vi "test New And Old Values Match.vi"(8 "error in (no error)":errorcluster, 11 "TestCase in":refnum<class "Routing and Faulting State Value Table Unit Tests.lvclass">) -> (0 "error out":errorcluster, 3 "TestCase out":refnum<class "Routing and Faulting State Value Table Unit Tests.lvclass">)   [LabVIEW 2019, in "Routing and Faulting State Value Table Unit Tests.lvclass"]
uses:
  Routing and Faulting State Value Table Unit Tests.lvclass
  Shared/Channel States.ctl
  Shared/Routing State.ctl
  Shared/Connection.ctl
  System Explorer/State-Value Row.ctl
  Routing and Faulting State Value Table Unit Tests.lvclass/Routing and Faulting State Value Table Unit Tests.ctl
  <vilib>/addons/_JKI Toolkits/VI Tester/TestCase.llb/TestCase.lvclass
  System Explorer/Routing and Faulting System Explorer.lvlib
  Shared/Routing and Faulting Shared.lvlib
  Scripting/Routing and Faulting Scripting.lvlib
  C:/Program Files (x86)/National Instruments/LabVIEW 2019/vi.lib/addons/_JKI Toolkits/VI Tester/TestCase.llb/TestCase.lvclass
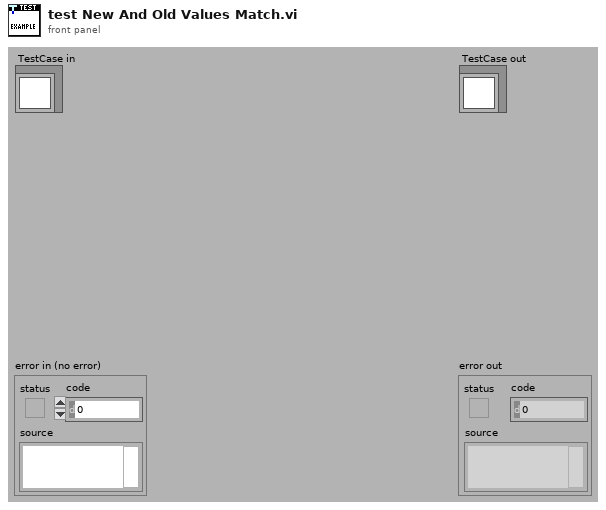
[diagram p1: front panel]
types:
  T1 = typedef "Routing and Faulting System Explorer.lvlib/State-Value Row.ctl" = cluster{"State":string, "State Value":string}
  T2 = typedef "Routing and Faulting Shared.lvlib/Channel States.ctl" = T3[]
  T3 = typedef "Routing and Faulting Shared.lvlib/Routing State.ctl" = cluster{"Name":string, "Description":string, "Value":i32, "Connection List":T4[]}
  T4 = typedef "Routing and Faulting Shared.lvlib/Connection.ctl" = cluster{"Module":string, "Source":string, "Destination":string}
  T5 = typedef "Custom Device API.lvlib/Custom Device Item Ref.ctl" = u64
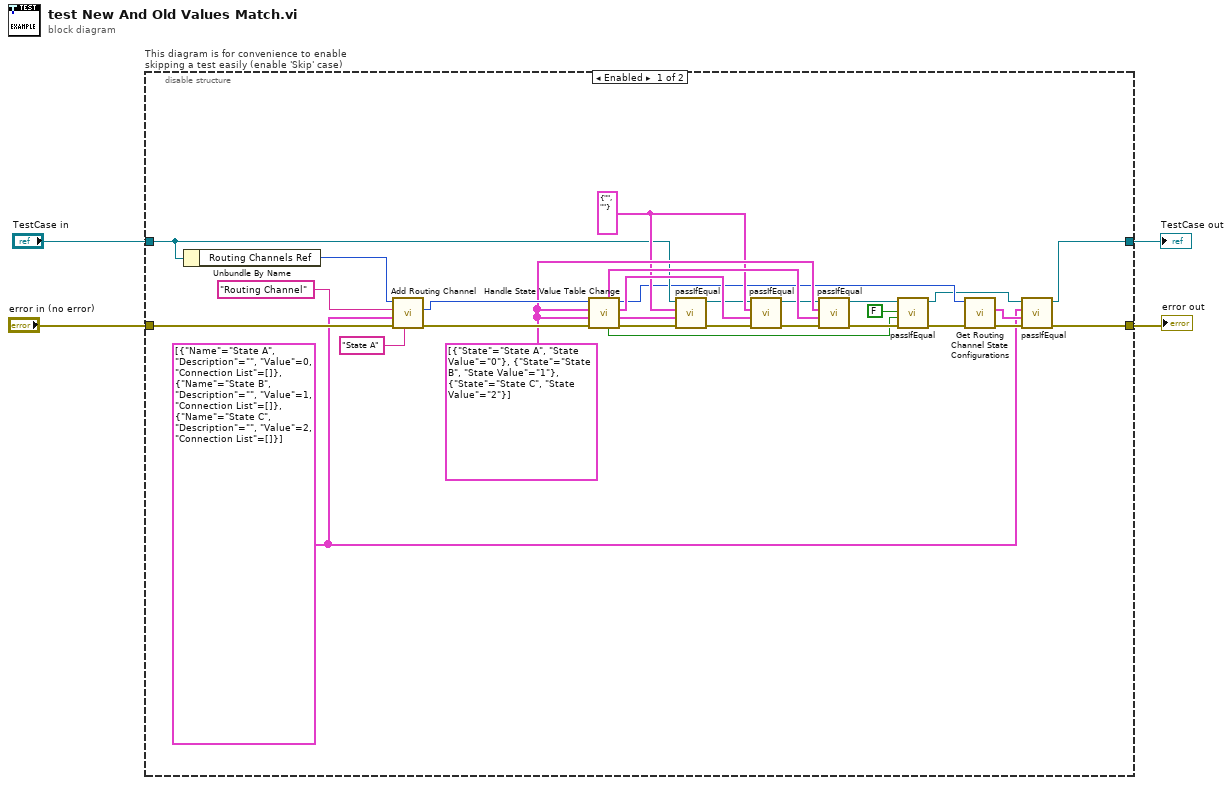
[diagram p0: block diagram]
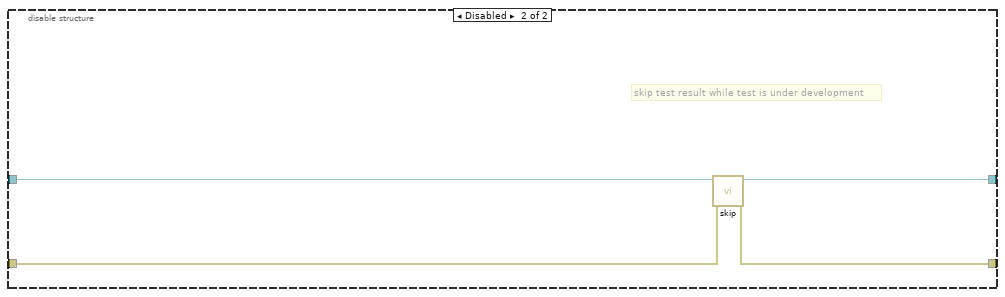
[diagram p2: hidden frame]
diagram:
  n1 = disable-structure "This diagram is for convenience to enable skipping a test easily (enable 'Skip' case)" shown="Enabled" {
    disable-tunnel: "TestCase in" -> [w13 w37]
    disable-tunnel: [w7 w35] -> w1
    disable-tunnel: [w9 w36] -> w3
    disable-tunnel: "error in (no error)" -> [w33 w34]
    frame Enabled {
      w16 = T1 {"State"="", "State Value"=""} ("old modified state and value")
      w17 = T1[] [{"State"="State A", "State Value"="0"}, {"State"="State B", "State Value"="1"}, {"State"="State C", "State Value"="2"}] ("NewVal")
      w5 = T2 [{"Name"="State A", "Description"="", "Value"=0, "Connection List"=[]}, {"Name"="State B", "Description"="", "Value"=1, "Connection List"=[]}, {"Name"="State C", "Description"="", "Value"=2, "Connection List"=[]}] ("state configurations")
      n2 = Unbundle By Name(w13) -> ("Routing Channels Ref"=w31:T5)
      n3 = call "Add Routing Channel.vi"("initial state"="State A", "error in"=w33, "state configurations"=w5, "channel name"="Routing Channel", "routing channels in"=w31) -> ("error out"=w32:errorcluster, "routing channel"=w26:T5)  [unwired: 4 in, 1 out]
      n4 = call "Handle State Value Table Change.vi"("error in (no error)"=w32, "OldVal"=w17, "NewVal"=w17, "routing channel in"=w26) -> ("error out"=w21:errorcluster, "old modified state and value"=w22:T1, "new modified state and value"=w24:T1, "routing channel out"=w12:T5, "update controls"=w19:bool, "coerced newval"=w29:T1[])  [unwired: 2 in]
      n5 = call-dynamic "passIfEqual.vi"("error in (no error)"=w21, "y"=w22, "x"=w16, "TestCase in"=w13) -> ("error out"=w23:errorcluster, "TestCase out"=w14:refnum<class "Routing and Faulting State Value Table Unit Tests.lvclass">)  [unwired: 6 in]
      n6 = call-dynamic "passIfEqual.vi"("error in (no error)"=w23, "y"=w24, "x"=w16, "TestCase in"=w14) -> ("error out"=w25:errorcluster, "TestCase out"=w15:refnum<class "Routing and Faulting State Value Table Unit Tests.lvclass">)  [unwired: 6 in]
      n7 = call-dynamic "passIfEqual.vi"("error in (no error)"=w25, "y"=w29, "x"=w17, "TestCase in"=w15) -> ("error out"=w30:errorcluster, "TestCase out"=w20:refnum<class "Routing and Faulting State Value Table Unit Tests.lvclass">)  [unwired: 6 in]
      n8 = call-dynamic "passIfEqual.vi"("error in (no error)"=w30, "y"=w19, "x"=FALSE ("update controls"), "TestCase in"=w20) -> ("error out"=w11:errorcluster, "TestCase out"=w8:refnum<class "Routing and Faulting State Value Table Unit Tests.lvclass">)  [unwired: 6 in]
      n9 = call "Get Routing Channel State Configurations.vi"("error in"=w11, "routing channel in"=w12) -> ("error out"=w10:errorcluster, "state configurations"=w6:T2)  [unwired: 7 in, 1 out]
      n10 = call-dynamic "passIfEqual.vi"("error in (no error)"=w10, "y"=w6, "x"=w5, "TestCase in"=w8) -> ("error out"=w9:errorcluster, "TestCase out"=w7:refnum<class "Routing and Faulting State Value Table Unit Tests.lvclass">)  [unwired: 6 in]
    }
    frame Disabled {
      # "skip test result while test is under development"
      n11 = call <vilib>:"skip.vi"("error in (no error)"=w34, "TestCase in"=w37) -> ("error out"=w36:errorcluster, "TestCase out"=w35:refnum<class "Routing and Faulting State Value Table Unit Tests.lvclass">)  [unwired: 8 in]
    }
  }
  "error out" <- w3
  "TestCase out" <- w1
